vi "Configure Devices.vi"(8 "error in":errorcluster, 11 "Device in":refnum<class "Device.lvclass">) -> (0 "error out":errorcluster, 3 "Device out":refnum<class "Device.lvclass">)   [LabVIEW 2014, in "DAQ Device.lvlib" / "Device.lvclass"]
uses:
  Device.lvclass
  <vilib>/ActorFramework/Actor/Actor.lvclass/Actor.ctl
  Device.lvclass/Device.ctl
  DAQ Device/Cfg Msg.ctl
  Devices/Configurable Device/Configurable Device.lvclass/Configurable Device.ctl
  Controller/Messages/Device Configuration/Get Serialized Device Configuration MSG.lvclass/Get Serialized Device Configuration MSG.ctl
  <vilib>/ActorFramework/Message Enqueuer/Message Enqueuer.lvclass/Message Enqueuer.ctl
  Messages/Generic CVT Init/Generic Init CVT Message.lvclass/Generic Init CVT Message.ctl
  Messages/Generic CVT Init/Write DevID.vi
  Messages/Generic CVT Init/Write SP.vi
  Devices/Configurable Device/Read ID.vi
  Devices/Configurable Device/Accessors/Read Device Type.vi
  Devices/Configurable Device/Accessors/Read label.vi
  Devices/Configurable Device/Accessors/Read SN.vi
  Devices/Configurable Device/Read controller_.vi
  Devices/Configurable Device/Accessors/Read Addr.vi
  Devices/Configurable Device/Accessors/Read Model.vi
  Controller/Messages/Device Configuration/Write cfg cluster.vi
  <vilib>/ActorFramework/Message Priority Queue/Priority Enqueue.vi
  Controller/xGlobal Data.vi
  Devices/Configurable Device/Configurable Device.lvclass
  <vilib>/ActorFramework/Actor/Actor.lvclass
  <vilib>/ActorFramework/Message Enqueuer/Message Enqueuer.lvclass
  DAQ Device.lvlib
  Messages/Generic CVT Init/Generic Init CVT Message.lvclass
  Controller/Messages/Device Configuration/Get Serialized Device Configuration MSG.lvclass
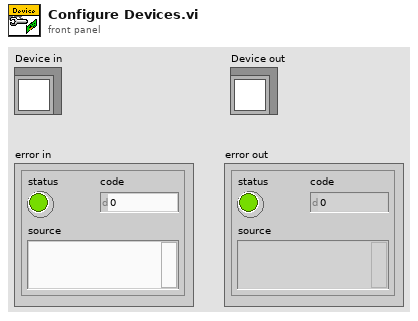
[diagram p1: front panel]
types:
  T1 = typedef "DAQ Device.lvlib/Cfg Msg.ctl" = cluster{"ID":string, "type":string, "label":string, "SN":string, "controller_":bool, "Addr":string, "Model":string}
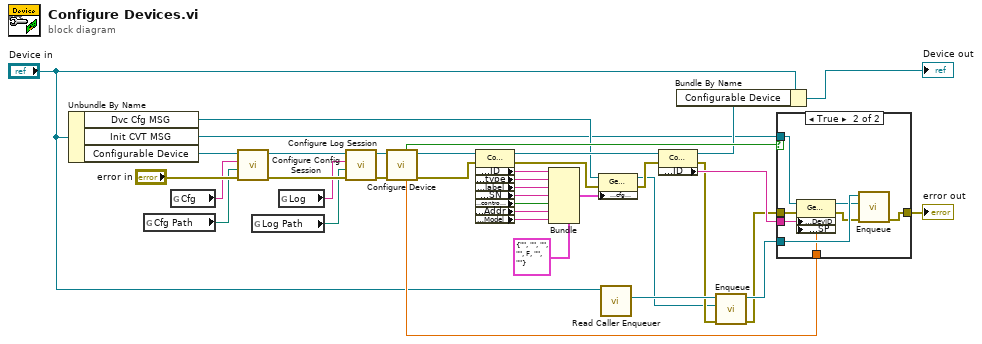
[diagram p0: block diagram]
diagram:
  n1 = Unbundle By Name("Device in") -> ("Dvc Cfg MSG"=w12:refnum<class "Get Serialized Device Configuration MSG.lvclass">, "Init CVT MSG"=w11:refnum<class "Generic Init CVT Message.lvclass">, "Configurable Device"=w10:refnum<class "Configurable Device.lvclass">)
  n2 = global read "xGlobal Data.vi" "Cfg Path"() -> (w2:path)
  n3 = global read "xGlobal Data.vi" "Cfg"() -> (w1:string)
  n4 = call "Configure Config Session.vi"("error in"="error in", "Path"=w2, "Ref Name"=w1, "Configurable Device in"=w10) -> ("error out"=w6:errorcluster, "Configurable Device out"=w9:refnum<class "Configurable Device.lvclass">)  [unwired: 6 in]
  n5 = global read "xGlobal Data.vi" "Log Path"() -> (w3:path)
  n6 = global read "xGlobal Data.vi" "Log"() -> (w4:string)
  n7 = call "Configure Log Session.vi"("error in"=w6, "Path"=w3, "Ref Name"=w4, "Configurable Device in"=w9) -> ("error out"=w5:errorcluster, "Configurable Device out"=w8:refnum<class "Configurable Device.lvclass">)  [unwired: 6 in]
  n8 = call-dynamic "Configure Device.vi"("error in"=w5, "Device in"=w8) -> ("error out"=w15:errorcluster, "Device out"=w28:refnum<class "Configurable Device.lvclass">, "SP"=w32:dbl, "Settable?"=w36:bool)  [unwired: 6 in]
  n9 = property class="Configurable Device"(reference=w28, error in=w15) -> (reference out=w17:refnum<class "Configurable Device.lvclass">, error out=w14:errorcluster, "Accessors:ID"=w27:string, "Accessors:type"=w26:string, "Accessors:label"=w25:string, "Accessors:SN"=w24:string, "Accessors:controller_"=w23:bool, "Accessors:Addr"=w22:string, "Accessors:Model"=w16:string)
  n10 = Bundle(cluster=T1 {"ID"="", "type"="", "label"="", "SN"="", "controller_"=FALSE, "Addr"="", "Model"=""}, "ID"=w27, "type"=w26, "label"=w25, "SN"=w24, "controller_"=w23, "Addr"=w22, "Model"=w16) -> (w20:T1)
  n11 = property class="Get Serialized Device Configura"(reference=w12, error in=w14, "Accessors:cfg cluster"=w20) -> (reference out=w18:refnum<class "Get Serialized Device Configuration MSG.lvclass">, error out=w19:errorcluster)
  n12 = call <vilib>:"Read Caller Enqueuer.vi"("Actor"="Device in") -> ("Caller Enqueuer"=w37:refnum<class "Message Enqueuer.lvclass">)  [unwired: 10 in]
  n13 = property class="Configurable Device"(reference=w17, error in=w19) -> (reference out=w34:refnum<class "Configurable Device.lvclass">, error out=w31:errorcluster, "Accessors:ID"=w33:string)
  n14 = Bundle By Name(cluster="Device in", "Configurable Device"=w34) -> (→"Device out":refnum<class "Device.lvclass">)
  n15 = call <vilib>:"Enqueue.vi"("error in (no error)"=w31, "Message"=w18, "Message Enqueuer in"=w37) -> ("error out"=w30:errorcluster, "Message Enqueuer out"=w35:refnum<class "Message Enqueuer.lvclass">)  [unwired: 7 in]
  n16 = case shown="True" w36 {
    tunnel: w35 -> [_ w47]
    tunnel: w11 -> [_ w46]
    tunnel: w33 -> [_ w45]
    tunnel: w32 -> [_ w44]
    tunnel: w30 -> [w39 w41]
    tunnel: [w39 w40] -> w29
    frame False {
    }
    frame True {
      n17 = property class="Generic Init CVT Message"(reference=w46, error in=w41, "Accessors:DevID"=w45, "Accessors:SP"=w44) -> (reference out=w43:refnum<class "Generic Init CVT Message.lvclass">, error out=w42:errorcluster)
      n18 = call <vilib>:"Enqueue.vi"("error in (no error)"=w42, "Message"=w43, "Message Enqueuer in"=w47) -> ("error out"=w40:errorcluster)  [unwired: 7 in, 1 out]
    }
  }
  "error out" <- w29
